vi "auto_alignment_v2-1.vi"() -> ()   [LabVIEW 2024]
uses:
  O:/DSG/Tyler/EIC/DIRC/daq/automated/Thorlabs.MotionControl.IntegratedStepperMotorsCLI.dll
  Thorlabs.MotionControl.IntegratedStepperMotorsCLI.dll
  O:/DSG/Tyler/EIC/DIRC/daq/automated/Thorlabs.MotionControl.Benchtop.StepperMotorCLI.dll
  Thorlabs.MotionControl.Benchtop.StepperMotorCLI.dll
  301acc45-ca86-4456-a934-959b204451cf.vi
  <vilib>/Array/Sort 2D Array - Pop Stack.vi
  <vilib>/Array/Sort 2D Array - Push Stack.vi
  301acc45-ca86-4456-a934-959b204451cf.vi/269d4b3b-47f5-49e3-8884-44851e4dd9d5.vi
  301acc45-ca86-4456-a934-959b204451cf.vi/6d99389c-673d-4efb-bf33-19b32bcf4cf8.vi
  <vilib>/Utility/file.llb/Read Delimited Spreadsheet (string).vi
  <vilib>/gmath/interp.llb/Interpolate 2D Scattered (1D).vi
  <vilib>/gmath/NI_AAL_Interpolation.lvlib
panel:
  out "sim_y-range":dbl[](array[numeric])
  out "sim_x-range":dbl[](array[numeric])
  out "sim_max":dbl[](array[numeric])
  out "Array":string[](array[string])
  in  "early-stop":bool
  out "state":string
  out "nPts":dbl
  out "pt-history":dbl[][](array[numeric])
  out "real-mode":bool
  out "sim-iCorr":dbl[](array[numeric])
  out "sim-pdy":dbl[](array[numeric])
  out "sim-pdx":dbl[](array[numeric])
  out "sim-data":dbl[][](array[numeric])
  out "Final Location":dbl[](array[numeric])
  in  "F=cRIO 2":bool
  out "x_c":dbl[](array[numeric])
  out "x_e":dbl[](array[numeric])
  out "x_r":dbl[](array[numeric])
  out "timeout":bool
  out "se_done":bool
  in  "se_goal":dbl=0.04
  out "squared_error":dbl
  out "x_o":dbl[](array[numeric])
  in  "F=cRIO":bool
  in  "xStart":dbl=265.0 format="%#_13g"
  in  "yStart":dbl=127.5 format="%#_13g"
  out "meter-error-out":errorcluster
  out "stage-error-out":errorcluster
  in  "stage-refs":T1
  in  "stage-error-in":errorcluster
  in  "meter-error-in":errorcluster
  in  "PD Values":cluster{"PD1":dbl, "PD2":dbl, "PD3":dbl}
  in  "nSamples":dbl=10.0 caption="# Samples"
  in  "meter-visa":refnum<visa-resource-name>
  in  "NM-params":T2={"alpha"=1.0, "gamma"=2.0, "rho"=0.5, "sigma"=0.5, "simplex L"=0.5}
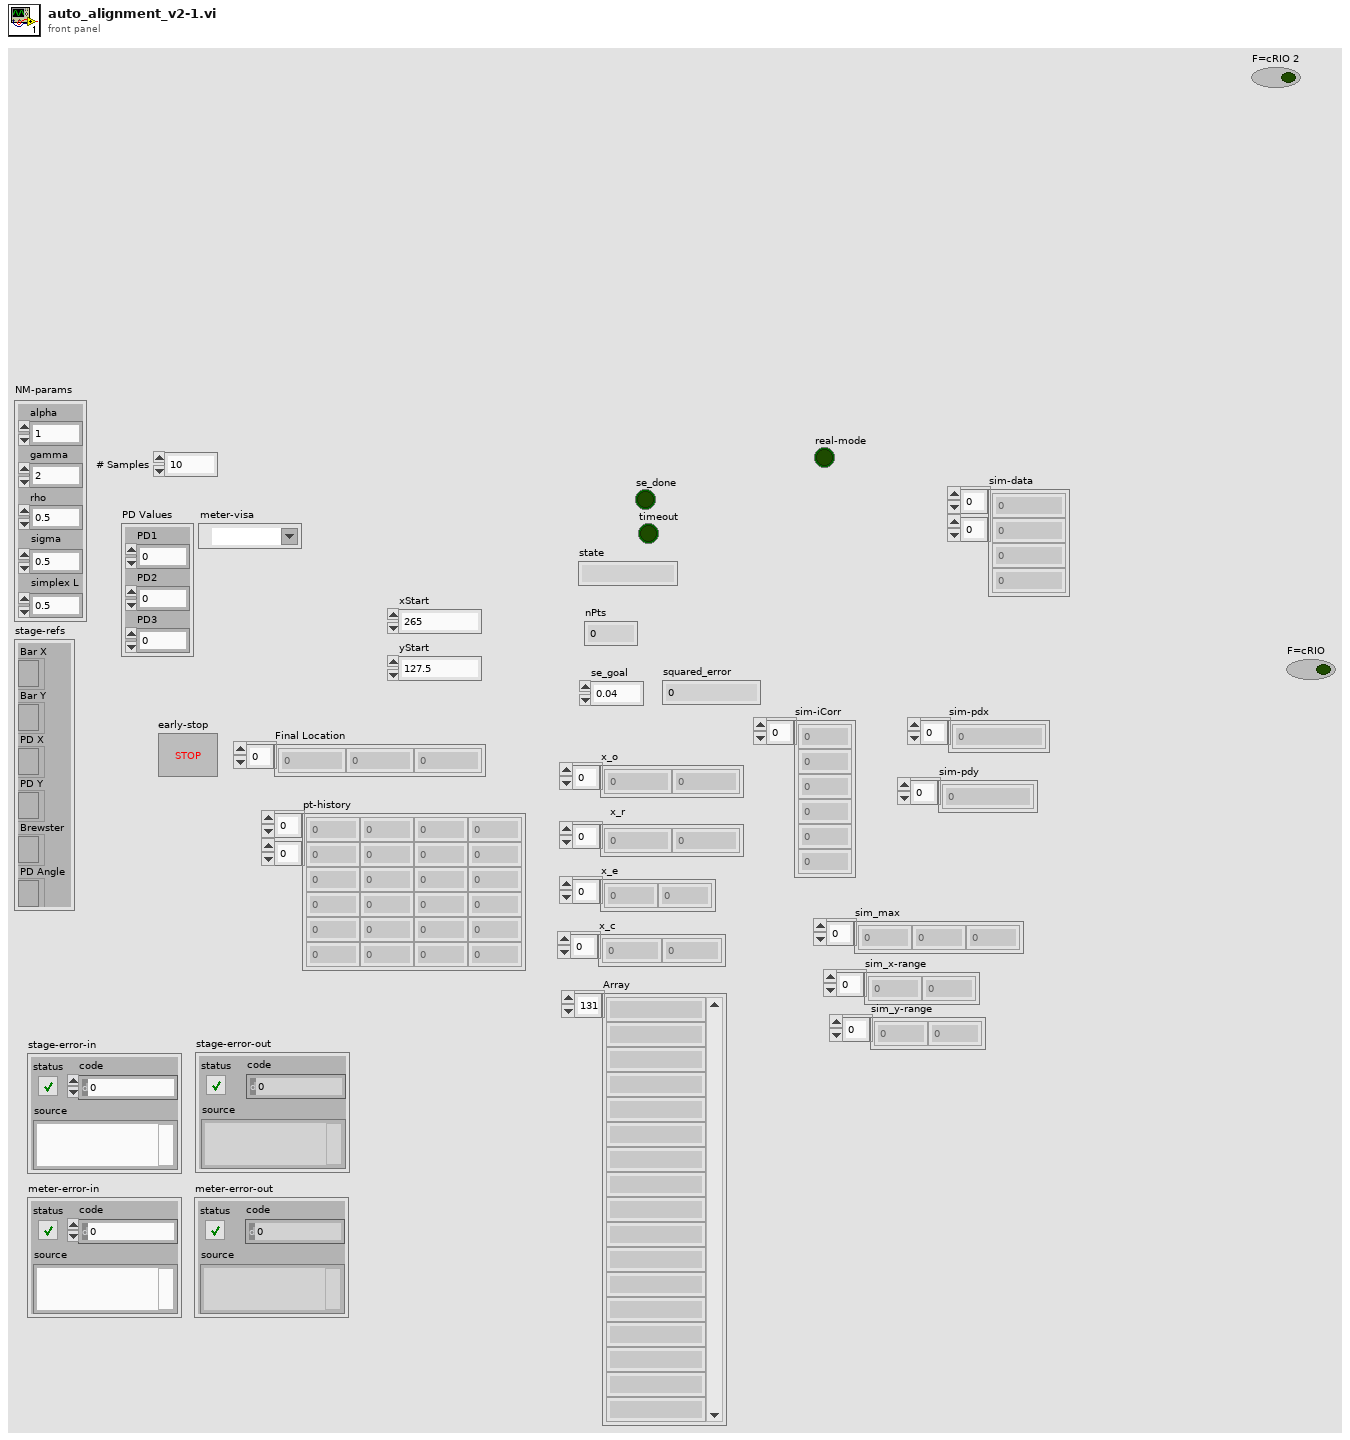
[diagram p1: front panel]
types:
  T1 = cluster{"Bar X":refnum<k24>, "Bar Y":refnum<k24>, "PD X":refnum<k24>, "PD Y":refnum<k24>, "Brewster":refnum<k24>, "PD Angle":refnum<k24>}
  T2 = cluster{"alpha":dbl, "gamma":dbl, "rho":dbl, "sigma":dbl, "simplex L":dbl}
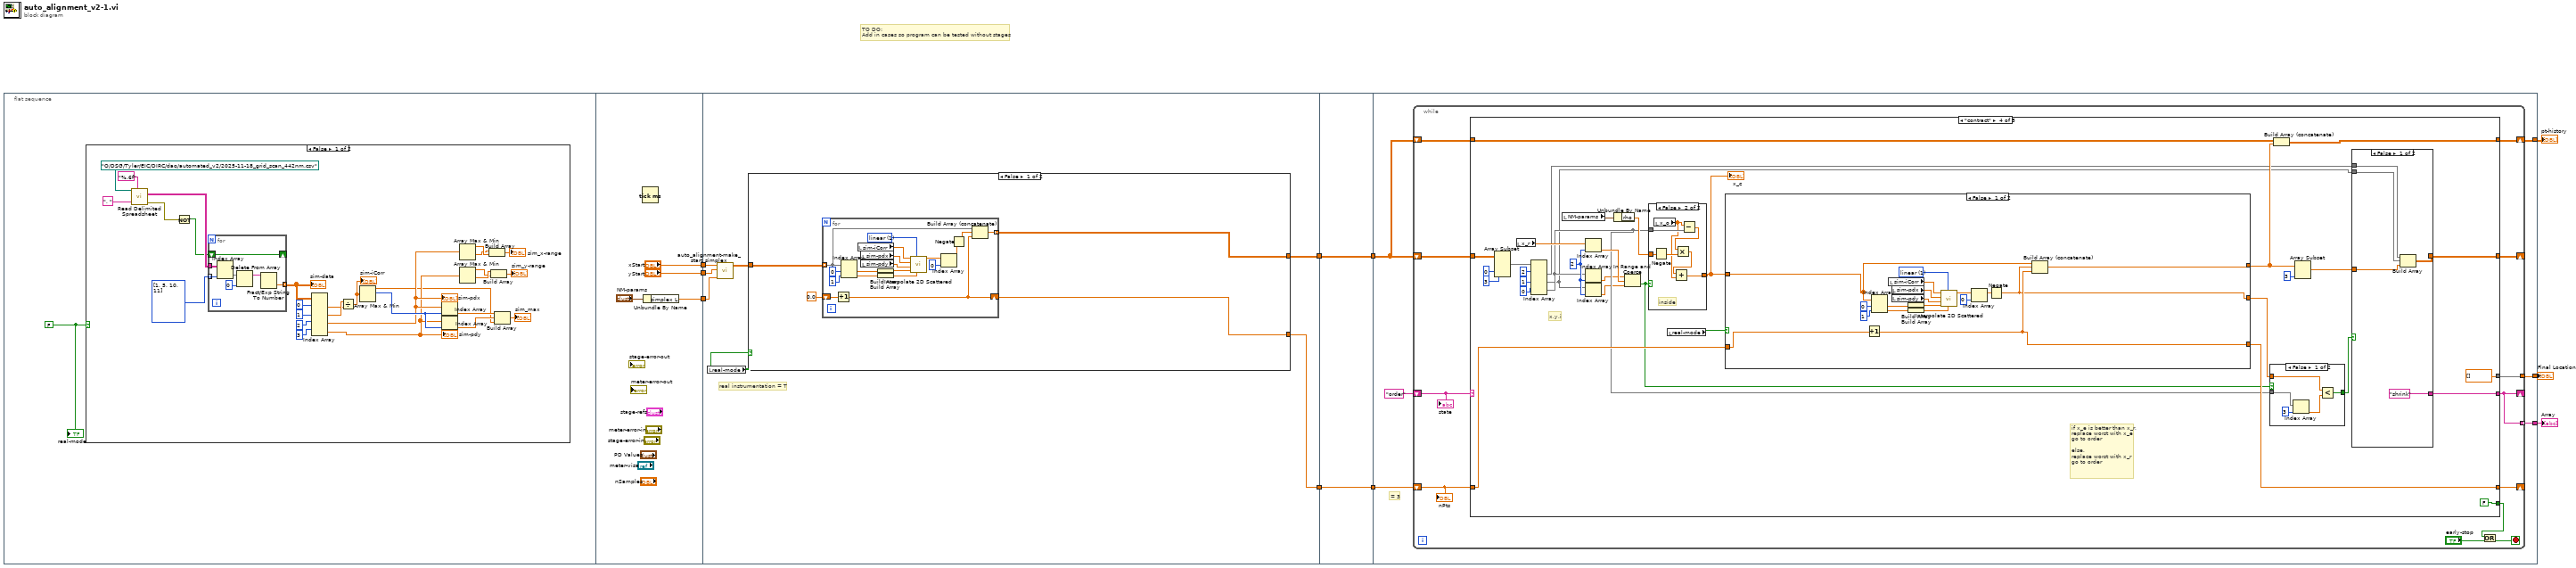
[diagram p0: block diagram]
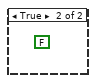
[diagram p2: hidden frame]
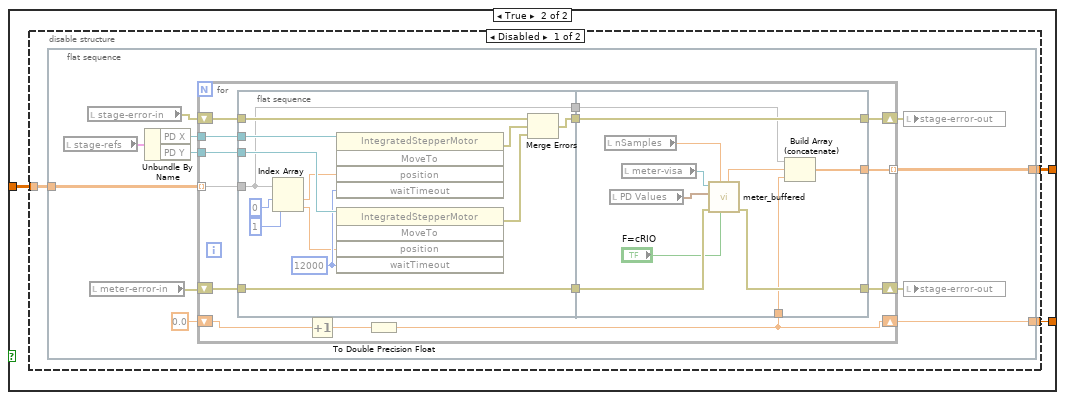
[diagram p3: hidden frame]
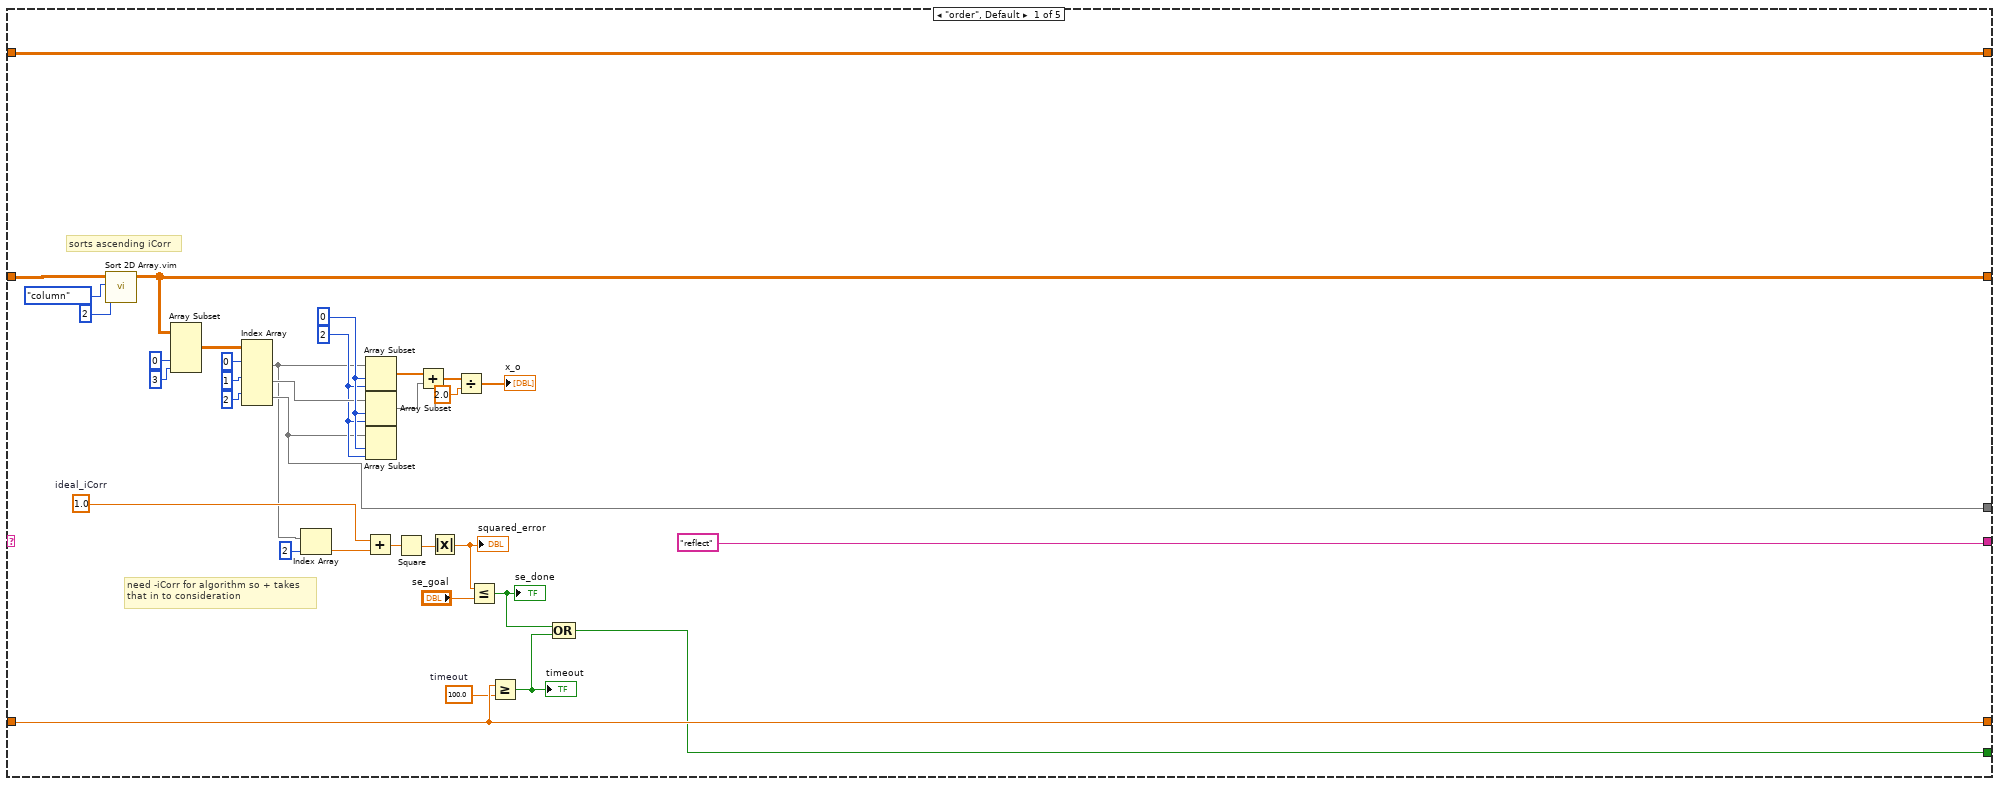
[diagram p5: hidden frame]
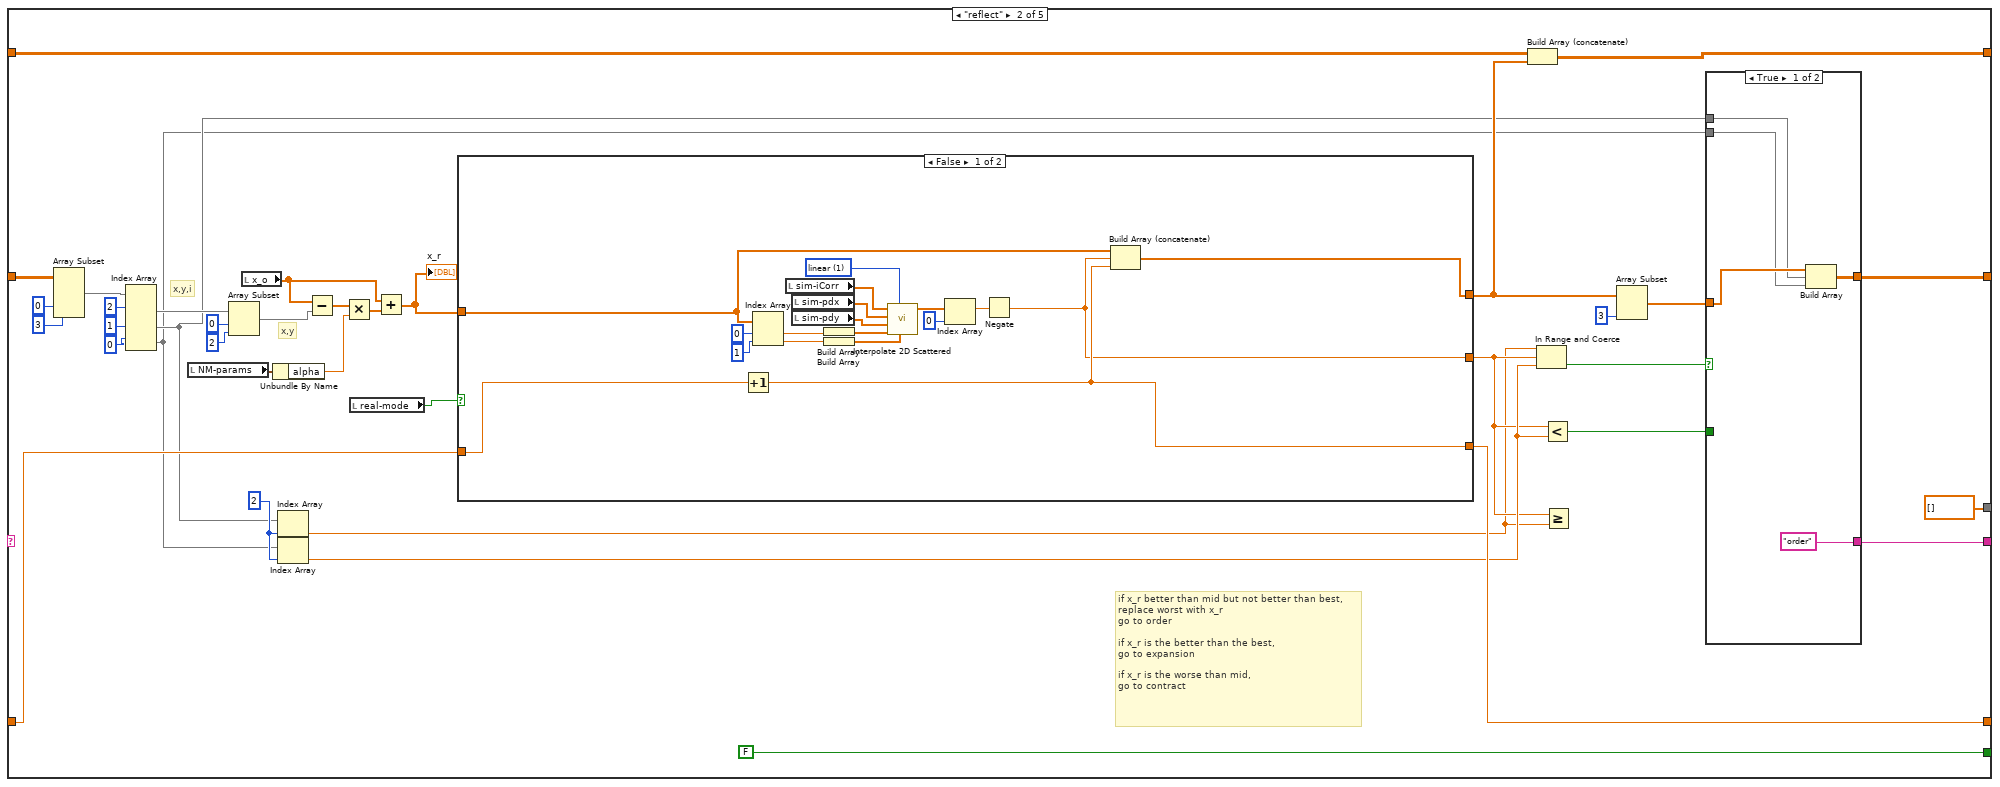
[diagram p6: hidden frame]
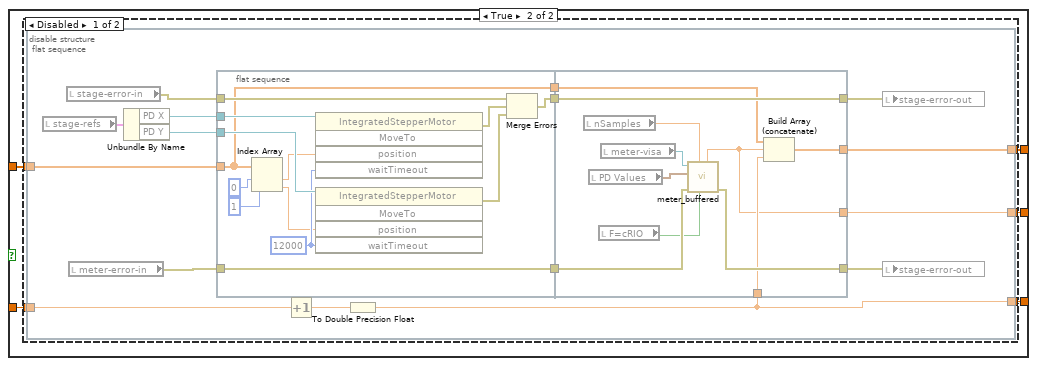
[diagram p7: hidden frame]
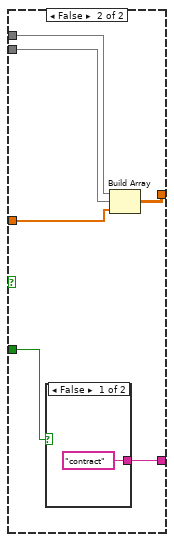
[diagram p9: hidden frame]
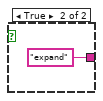
[diagram p10: hidden frame]
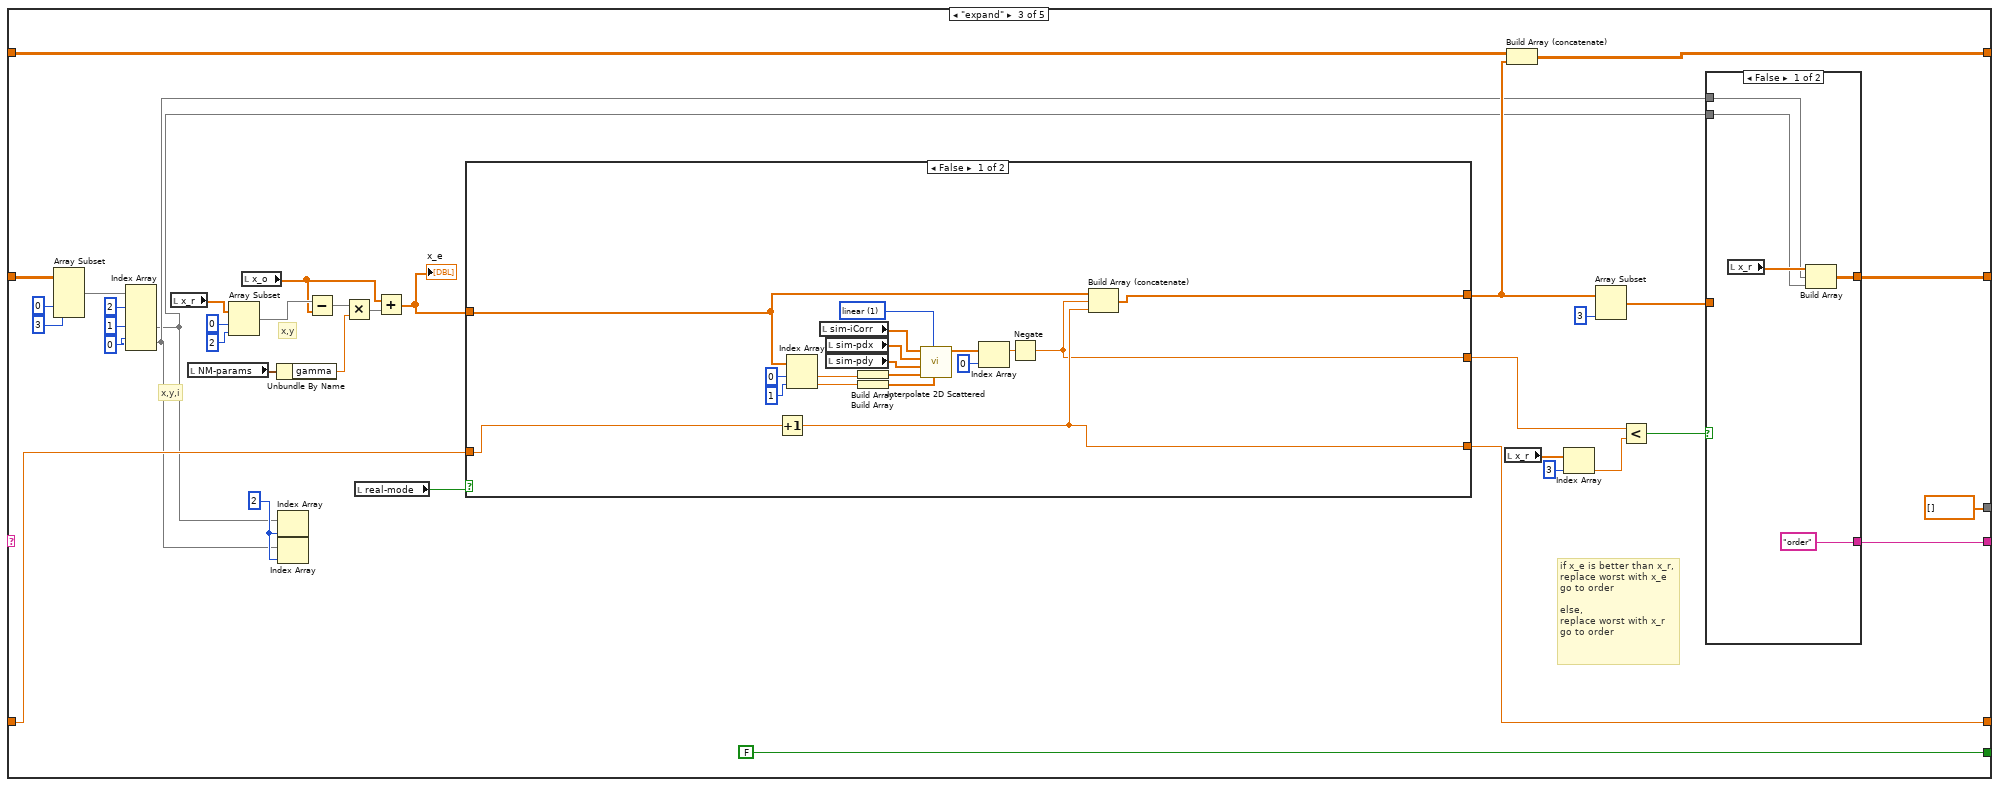
[diagram p11: hidden frame]
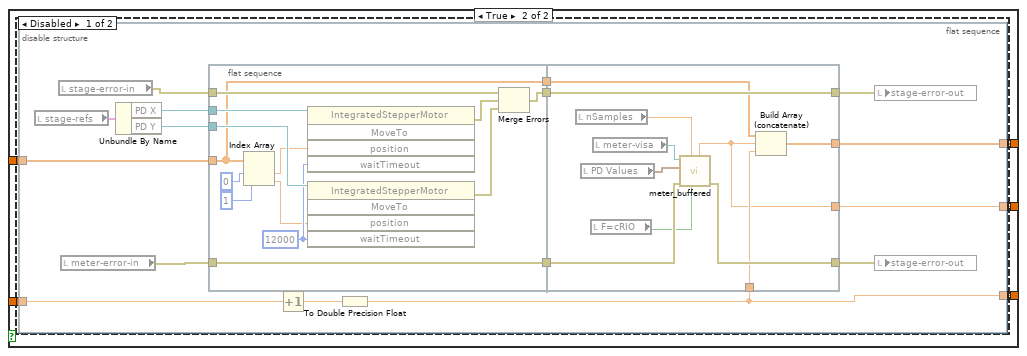
[diagram p12: hidden frame]
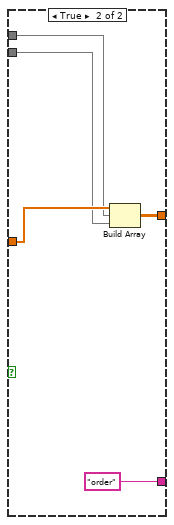
[diagram p14: hidden frame]
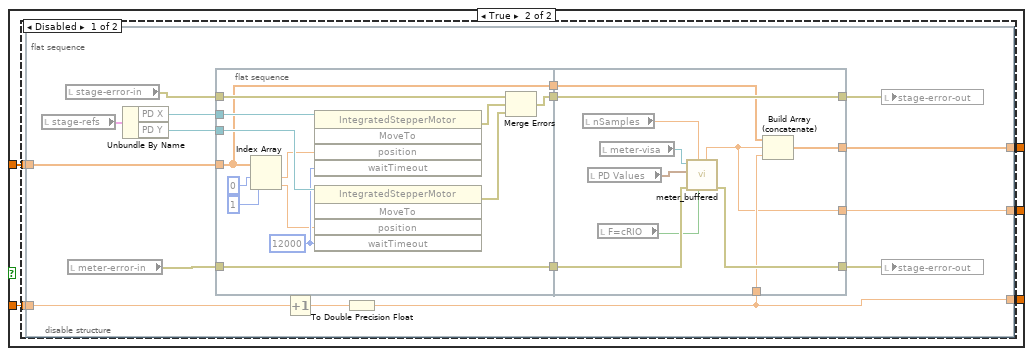
[diagram p15: hidden frame]
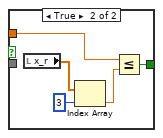
[diagram p17: hidden frame]
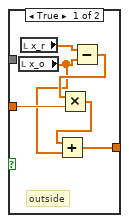
[diagram p18: hidden frame]
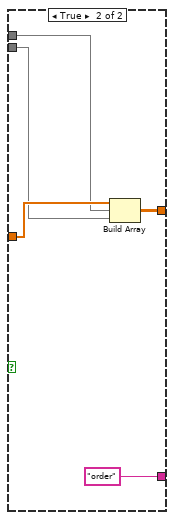
[diagram p19: hidden frame]
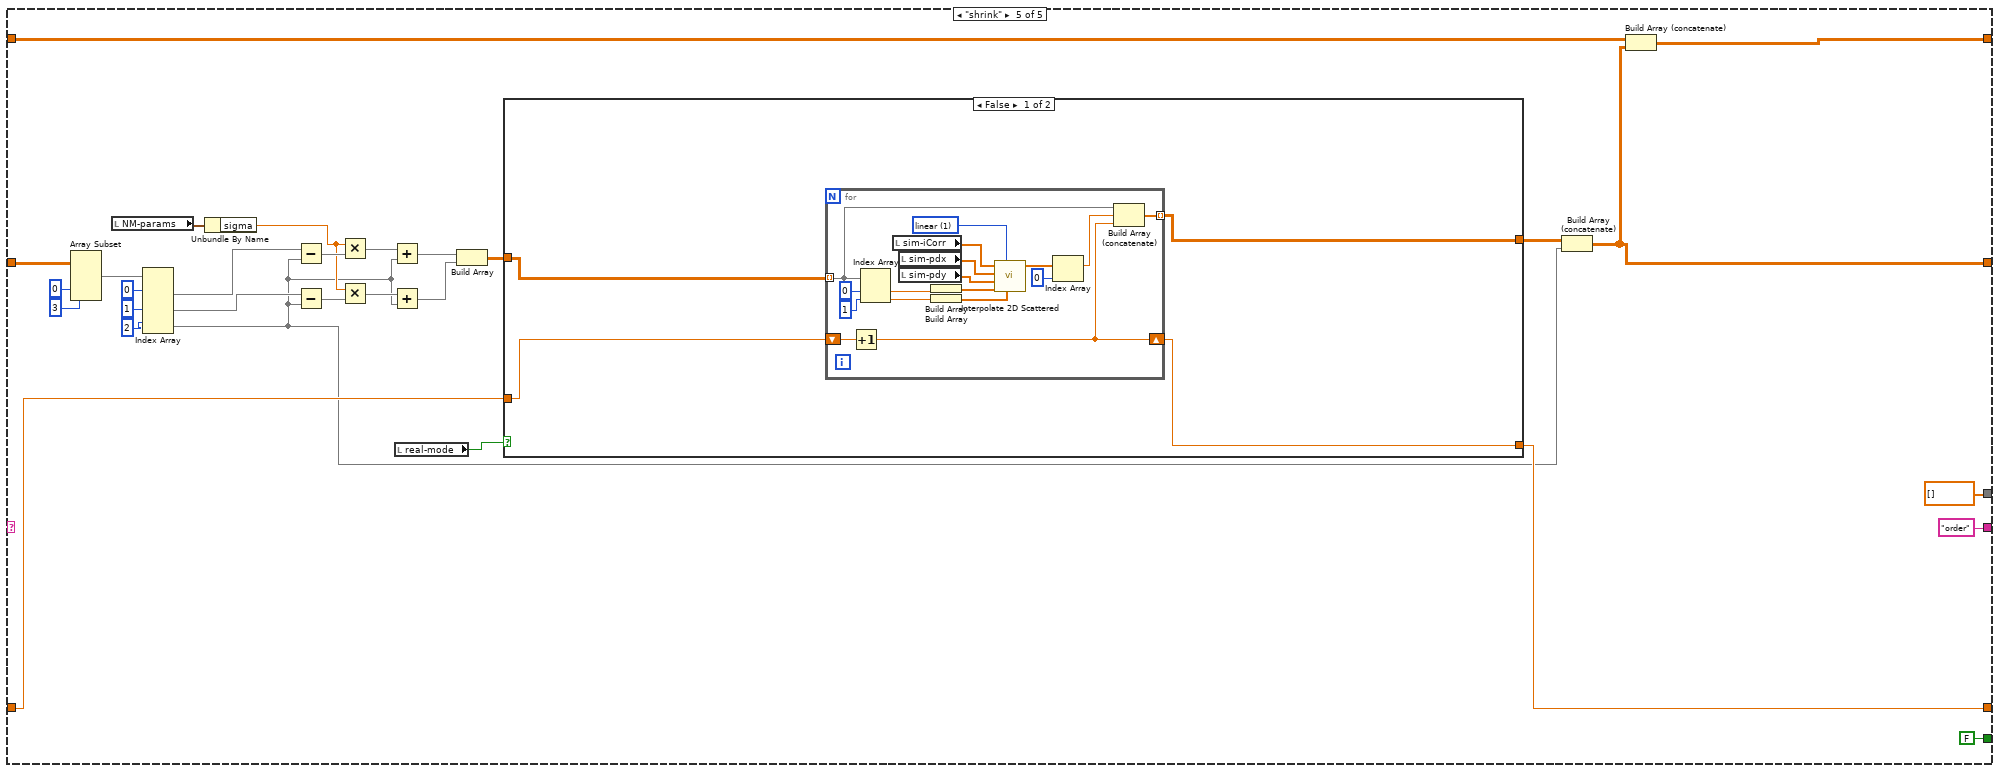
[diagram p20: hidden frame]
diagram:
  # "TO DO:\nAdd in cases so program can be tested without stages"
  n1 = flat-sequence {
    tunnel: ["xStart"] -> w10
    tunnel: ["yStart"] -> w9
    tunnel: [w47] -> w8
    tunnel: w10 -> [w53]
    tunnel: w9 -> [w54]
    tunnel: w8 -> [w55]
    tunnel: [w57] -> w4
    tunnel: [w56] -> w2
    tunnel: w4 -> [w136]
    tunnel: [w136] -> w3
    tunnel: w2 -> [w135]
    tunnel: [w135] -> w1
    tunnel: w3 -> [w140]
    tunnel: w1 -> [w141]
    tunnel: [w139] -> w7
    tunnel: [w138] -> w6
    tunnel: [w137] -> w5
    frame #0 {
      w11 = FALSE
      n2 = case shown="False" w11 {
        frame False {
          n3 = call-poly <vilib>:"Read Delimited Spreadsheet.vi"("file path (dialog if empty)"=path "O:/DSG/Tyler/EIC/DIRC/daq/automated_v2/2025-11-18_grid_scan_442nm.csv", "format (%s)"="%.6f" ("format (%.3f)"), "delimiter (\\t)"=", " ("delimiter (\\t)")) -> ("all rows"=w35:string[][], "error out"=w37:errorcluster)  [unwired: 7 in, 4 out]
          n4 = Not(x=w37) -> (.not. x?=w33:bool)
          n5 = for {
            tunnel: i32[] [1, 5, 10, 11] -> [w45] mode=indexing
            tunnel: w35 -> [w46]
            shift-right: [w44] -> _
            shift-left: w33 -> [w44]
            tunnel: [w40] -> w26 mode=indexing
            n6 = Index Array(array=w46, index (col)=w45) -> (element=w43:string[])  [unwired: 1 in]
            n7 = Delete From Array(array=w43, index=0) -> (array with subset deleted=w41:string[])  [unwired: 1 in, 1 out]
            n8 = Fract/Exp String To Number(string=w41) -> (number=w40:dbl[])  [unwired: 3 in, 1 out]
          }
          "sim-data" <- w26
          n9 = Index Array(array=w26, index (row) #1=0 ("index"), index (row) #2=1 ("index (row)"), index (row) #3=2 ("index (row)"), index (row) #4=3 ("index (row)")) -> (element #1=w27:dbl[], element #2=w28:dbl[], element #3=w21:dbl[], element #4=w20:dbl[])  [unwired: 4 in]
          "sim-pdx" <- w21
          "sim-pdy" <- w20
          n10 = Divide(x=w28, y=w27) -> (x/y=w12:dbl[])
          "sim-iCorr" <- w12
          n11 = Array Max & Min(array=w12) -> (max value=w13:dbl, max index (indices)=w25:i32)  [unwired: 2 out]
          n12 = Index Array(array=w21, index=w25) -> (element=w24:dbl)
          n13 = Index Array(array=w20, index=w25) -> (element=w23:dbl)
          n14 = Array Max & Min(array=w21) -> (max value=w19:dbl, min value=w18:dbl)  [unwired: 2 out]
          n15 = Array Max & Min(array=w20) -> (max value=w15:dbl, min value=w17:dbl)  [unwired: 2 out]
          n16 = Build Array(w18, w19) -> (→"sim_x-range":dbl[])
          n17 = Build Array(w17, w15) -> (→"sim_y-range":dbl[])
          n18 = Build Array(w24, w23, w13) -> (→"sim_max":dbl[])
        }
        frame True {
          (unwired) FALSE
        }
      }
      "real-mode" <- w11
    }
    frame #1 {
      n19 = Tick Count (ms)() -> ()  [unwired: 1 out]
      n20 = Unbundle By Name("NM-params") -> ("simplex L"=w47:dbl)
    }
    frame #2 {
      # "real instrumentation = T"
      n21 = local read "real-mode"() -> (w51:bool)
      n22 = call "auto_alignment-make_start_simplex.vi"("L"=w55, "yStart"=w54, "xStart"=w53) -> ("Array"=w52:dbl[][])  [unwired: 8 in]
      n23 = case shown="False" w51 {
        tunnel: [w58 w82] -> w57
        tunnel: [w60 w81] -> w56
        tunnel: w52 -> [w59 w80]
        frame False {
          n24 = for {
            shift-right: [w63] -> w60
            shift-left: 0.0 -> [w75]
            tunnel: w59 -> [w68] mode=indexing
            tunnel: [w67] -> w58 mode=indexing
            w79 = 1 items=["nearest", "linear", "cubic", "biharmonic spline "] ("method")
            n25 = Increment(x=w75) -> (x+1=w63:dbl)
            n26 = Index Array(array=w68, index #1=0 ("index"), index #2=1 ("index")) -> (element #1=w72:dbl, element #2=w70:dbl)
            n27 = local read "sim-iCorr"() -> (w78:dbl[])
            n28 = local read "sim-pdx"() -> (w77:dbl[])
            n29 = local read "sim-pdy"() -> (w76:dbl[])
            n30 = Build Array(w72) -> (w71:dbl[])
            n31 = Build Array(w70) -> (w69:dbl[])
            n32 = call-poly <vilib>:"Interpolate 2D Scattered.vi"("Yi"=w69, "method"=w79, "Xi"=w71, "Y"=w76, "X"=w77, "Z"=w78) -> ("Zi"=w66:dbl[])  [unwired: 4 in, 1 out]
            n33 = Index Array(array=w66, index=0) -> (element=w65:dbl)
            n34 = Negate(x=w65) -> (-x=w62:dbl)
            n35 = Build Array (concatenate)(w68, w62, w63) -> (w67:dbl[])
          }
        }
        frame True {
          n36 = disable-structure shown="Disabled" {
            disable-tunnel: [w85 _] -> w82
            disable-tunnel: [w84 _] -> w81
            disable-tunnel: w80 -> [w83 _]
            frame Disabled {
              n37 = flat-sequence {
                tunnel: [w94] -> w85
                tunnel: [w88] -> w84
                tunnel: w83 -> [w86]
                frame #0 {
                  n38 = local read "stage-refs"() -> (w90:T1)
                  n39 = local read "stage-error-in"() -> (w91:errorcluster)
                  n40 = local read "meter-error-in"() -> (w89:errorcluster)
                  n41 = Unbundle By Name(w90) -> ("PD X"=w96:refnum<k24>, "PD Y"=w95:refnum<k24>)
                  n42 = for {
                    tunnel: w96 -> [w110]
                    tunnel: w95 -> [w109]
                    tunnel: w86 -> [w106] mode=indexing
                    shift-right: [w104] -> w92
                    shift-left: w91 -> [w108]
                    tunnel: [w107] -> w94 mode=indexing
                    shift-right: [w105] -> w93
                    shift-left: w89 -> [w103]
                    shift-right: [w98] -> w88
                    shift-left: 0.0 -> [w97]
                    n43 = flat-sequence {
                      tunnel: w110 -> [w121]
                      tunnel: w109 -> [w120]
                      tunnel: w108 -> [w114]
                      tunnel: w106 -> [w112]
                      tunnel: w103 -> [w111]
                      tunnel: [w113] -> w102
                      tunnel: [w112] -> w101
                      tunnel: [w111] -> w100
                      tunnel: [w134] -> w104
                      tunnel: [w130] -> w105
                      tunnel: [w133] -> w107
                      tunnel: w102 -> [w134]
                      tunnel: w101 -> [w132]
                      tunnel: w100 -> [w131]
                      tunnel: w98 -> [w124]
                      frame #0 {
                        w119 = 12000 ("waitTimeout")
                        n44 = Index Array(array=w112, index #1=0 ("index"), index #2=1 ("index")) -> (element #1=w116:dbl, element #2=w115:dbl)
                        n45 = invoke class="IntegratedStepperMotor" method="MoveTo"(reference=w121, "position"=w116, "waitTimeout"=w119) -> (error out=w123:errorcluster)  [unwired: 2 in, 4 out]
                        n46 = invoke class="IntegratedStepperMotor" method="MoveTo"(reference=w120, "position"=w115, "waitTimeout"=w119) -> (error out=w122:errorcluster)  [unwired: 2 in, 4 out]
                        n47 = Merge Errors(w114, w123, w122) -> (w113:errorcluster)
                      }
                      frame #1 {
                        n48 = local read "nSamples"() -> (w129:dbl)
                        n49 = local read "PD Values"() -> (w127:cluster{"PD1":dbl, "PD2":dbl, "PD3":dbl})
                        n50 = local read "meter-visa"() -> (w128:refnum<visa-resource-name>)
                        n51 = call "meter_buffered.vi"("F=cRIO"="F=cRIO", "Samples"=w129, "error in"=w131, "PD ranges"=w127, "meter-VISA"=w128) -> ("error out"=w130:errorcluster, "iCorr"=w125:dbl)  [unwired: 2 in, 3 out]
                        n52 = Build Array (concatenate)(w132, w125, w124) -> (w133:dbl[])
                      }
                    }
                    n53 = Increment(x=w97) -> (x+1=w99:dbl)
                    n54 = To Double Precision Float(number=w99) -> (double precision float=w98:dbl)
                  }
                  n55 = local write "stage-error-out"(w92) -> ()
                  n56 = local write "stage-error-out"(w93) -> ()
                }
              }
            }
            frame Enabled {
            }
          }
        }
      }
    }
    frame #3 {
    }
    frame #4 {
      # "= 3"
      n57 = while {
        shift-right: [w148] -> w138
        shift-left: w140 -> [w153]
        shift-right: [w149] -> _
        shift-left: w140 -> [w152]
        shift-right: [w143] -> _
        shift-left: "order" -> [w154]
        shift-right: [w150] -> _
        shift-left: w141 -> [w151]
        tunnel: [w147] -> w139
        tunnel: [w143] -> w137 mode=indexing
        stop <- w145 stop-if-true
        n58 = case shown="\"contract\"" w154 {
          tunnel: w153 -> [w174 w207 w327 w444 w563]
          tunnel: w152 -> [w172 w192 w324 w442 w576]
          tunnel: ["reflect" w203 w322 w440 "order"] -> w143
          tunnel: w151 -> [w163 w209 w329 w446 w564]
          tunnel: [w163 w208 w328 w445 w561] -> w150
          tunnel: [w164 w204 w323 w441 w557] -> w149
          tunnel: [w159 FALSE FALSE FALSE FALSE] -> w144
          tunnel: [w174 w206 w326 w443 w562] -> w148
          tunnel: [w158 dbl[] [] dbl[] [] dbl[] [] dbl[] []] -> w147
          frame "order", Default {
            w162 = 100.0  # timeout
            w169 = 1.0  # ideal_iCorr
            w179 = 2 ("length")
            w181 = 0 ("index")
            # "need -iCorr for algorithm so + takes\nthat in to consideration"
            # "sorts ascending iCorr"
            n59 = call "Sort 2D Array.vim"("index"=2, "dimension to index (column)"=enum16{"column", "row"}."column", "2D array"=w172) -> ("sorted 2D array"=w164:dbl[][])  [unwired: 7 in, 1 out]
            n60 = Array Subset(array=w164, index (col)=0 ("index"), length (col)=3 ("length")) -> (w173:dbl[][])  [unwired: 2 in]
            n61 = Index Array(array=w173, index (row) #1=0 ("index (row)"), index (row) #2=1 ("index (row)"), index (row) #3=2 ("index (row)")) -> (element #1=w155:dbl[], element #2=w180:dbl[], element #3=w158:dbl[])  [unwired: 3 in]
            n62 = Index Array(array=w155, index=2) -> (element=w170:dbl)
            n63 = Add(x=w169, y=w170) -> (x+y=w168:dbl)
            n64 = Array Subset(array=w155, index=w181, length=w179) -> (w157:dbl[])
            n65 = Array Subset(array=w180, index=w181, length=w179) -> (w156:dbl[])
            n66 = Array Subset(array=w158, index=w181, length=w179) -> ()  [unwired: 1 out]
            n67 = Square(x=w168) -> (x^2=w167:dbl)
            n68 = Add(x=w157, y=w156) -> (x+y=w178:dbl[])
            n69 = Absolute Value(x=w167) -> (abs(x)=w166:dbl)
            "squared_error" <- w166
            n70 = Divide(x=w178, y=2.0) -> (x/y=→"x_o":dbl[])
            n71 = Less Or Equal?(x=w166, y="se_goal") -> (x <= y?=w161:bool)
            "se_done" <- w161
            n72 = Greater Or Equal?(x=w163, y=w162) -> (x >= y?=w160:bool)
            "timeout" <- w160
            n73 = Compound Arithmetic op=OR(w161, w160) -> (w159:bool)
          }
          frame "reflect" {
            w205 = 2 ("index")
            # "x,y"
            # "if x_r better than mid but not better than best, \nreplace worst with x_r\ngo to order\n\nif x_r is the better than the best,\ngo to expansion\n\nif x_r is the worse than mid,\ngo to contract"
            # "x,y,i"
            n74 = Array Subset(array=w192, index (col)=0 ("index"), length (col)=3 ("length")) -> (w191:dbl[][])  [unwired: 2 in]
            n75 = Index Array(array=w191, index (row) #1=2 ("index (row)"), index (row) #2=1 ("index (row)"), index (row) #3=0 ("index (row)")) -> (element #1=w219:dbl[], element #2=w190:dbl[], element #3=w189:dbl[])  [unwired: 3 in]
            n76 = local read "NM-params"() -> (w216:T2)
            n77 = Array Subset(array=w219, index=0 ("index (row)"), length=2 ("index (row)")) -> (w215:dbl[])
            n78 = local read "x_o"() -> (w212:dbl[])
            n79 = Unbundle By Name(w216) -> ("alpha"=w213:dbl)
            n80 = Index Array(array=w190, index=w205) -> (element=w194:dbl)
            n81 = Index Array(array=w189, index=w205) -> (element=w197:dbl)
            n82 = Subtract(x=w212, y=w215) -> (x-y=w214:dbl[])
            n83 = Multiply(x=w214, y=w213) -> (x*y=w211:dbl[])
            n84 = local read "real-mode"() -> (w198:bool)
            n85 = Add(x=w212, y=w211) -> (x+y=w210:dbl[])
            "x_r" <- w210
            n86 = case shown="False" w198 {
              tunnel: w210 -> [w231 w248]
              tunnel: w209 -> [w230 w247]
              tunnel: [w229 w246] -> w208
              tunnel: [w226 w245] -> w195
              tunnel: [w227 w244] -> w202
              frame False {
                w243 = 1 items=["nearest", "linear", "cubic", "biharmonic spline "] ("method")
                n87 = Increment(x=w230) -> (x+1=w229:dbl)
                n88 = Index Array(array=w231, index #1=0 ("index"), index #2=1 ("index")) -> (element #1=w237:dbl, element #2=w235:dbl)
                n89 = local read "sim-iCorr"() -> (w242:dbl[])
                n90 = local read "sim-pdx"() -> (w241:dbl[])
                n91 = local read "sim-pdy"() -> (w240:dbl[])
                n92 = Build Array(w237) -> (w236:dbl[])
                n93 = Build Array(w235) -> (w234:dbl[])
                n94 = call-poly <vilib>:"Interpolate 2D Scattered.vi"("Yi"=w234, "method"=w243, "Xi"=w236, "Y"=w240, "X"=w241, "Z"=w242) -> ("Zi"=w233:dbl[])  [unwired: 4 in, 1 out]
                n95 = Index Array(array=w233, index=0) -> (element=w228:dbl)
                n96 = Negate(x=w228) -> (-x=w226:dbl)
                n97 = Build Array (concatenate)(w231, w226, w229) -> (w227:dbl[])
              }
              frame True {
                n98 = disable-structure shown="Disabled" {
                  disable-tunnel: w248 -> [w253 _]
                  disable-tunnel: w247 -> [w252 _]
                  disable-tunnel: [w251 _] -> w246
                  disable-tunnel: [w250 _] -> w245
                  disable-tunnel: [w249 _] -> w244
                  frame Disabled {
                    n99 = flat-sequence {
                      tunnel: [w267] -> w249
                      tunnel: [w261] -> w251
                      tunnel: w253 -> [w260]
                      tunnel: w252 -> [w255]
                      tunnel: [w254] -> w250
                      frame #0 {
                        n100 = local read "stage-refs"() -> (w263:T1)
                        n101 = local read "stage-error-in"() -> (w264:errorcluster)
                        n102 = local read "meter-error-in"() -> (w262:errorcluster)
                        n103 = Unbundle By Name(w263) -> ("PD X"=w269:refnum<k24>, "PD Y"=w268:refnum<k24>)
                        n104 = flat-sequence {
                          tunnel: w269 -> [w280]
                          tunnel: w268 -> [w279]
                          tunnel: w264 -> [w273]
                          tunnel: w260 -> [w271]
                          tunnel: w262 -> [w270]
                          tunnel: [w272] -> w259
                          tunnel: [w271] -> w258
                          tunnel: [w270] -> w257
                          tunnel: [w293] -> w265
                          tunnel: [w289] -> w266
                          tunnel: [w292] -> w267
                          tunnel: w259 -> [w293]
                          tunnel: w258 -> [w291]
                          tunnel: w257 -> [w290]
                          tunnel: w261 -> [w285]
                          tunnel: [w284] -> w254
                          frame #0 {
                            w278 = 12000 ("waitTimeout")
                            n105 = Index Array(array=w271, index #1=0 ("index"), index #2=1 ("index")) -> (element #1=w275:dbl, element #2=w274:dbl)
                            n106 = invoke class="IntegratedStepperMotor" method="MoveTo"(reference=w280, "position"=w275, "waitTimeout"=w278) -> (error out=w282:errorcluster)  [unwired: 2 in, 4 out]
                            n107 = invoke class="IntegratedStepperMotor" method="MoveTo"(reference=w279, "position"=w274, "waitTimeout"=w278) -> (error out=w281:errorcluster)  [unwired: 2 in, 4 out]
                            n108 = Merge Errors(w273, w282, w281) -> (w272:errorcluster)
                          }
                          frame #1 {
                            n109 = local read "nSamples"() -> (w288:dbl)
                            n110 = local read "PD Values"() -> (w286:cluster{"PD1":dbl, "PD2":dbl, "PD3":dbl})
                            n111 = local read "F=cRIO"() -> (w283:bool)
                            n112 = local read "meter-visa"() -> (w287:refnum<visa-resource-name>)
                            n113 = call "meter_buffered.vi"("F=cRIO"=w283, "Samples"=w288, "error in"=w290, "PD ranges"=w286, "meter-VISA"=w287) -> ("error out"=w289:errorcluster, "iCorr"=w284:dbl)  [unwired: 2 in, 3 out]
                            n114 = Build Array (concatenate)(w291, w284, w285) -> (w292:dbl[])
                          }
                        }
                        n115 = Increment(x=w255) -> (x+1=w256:dbl)
                        n116 = To Double Precision Float(number=w256) -> (double precision float=w261:dbl)
                        n117 = local write "stage-error-out"(w265) -> ()
                        n118 = local write "stage-error-out"(w266) -> ()
                      }
                    }
                  }
                  frame Enabled {
                  }
                }
              }
            }
            n119 = Build Array (concatenate)(w207, w202) -> (w206:dbl[][])
            n120 = In Range and Coerce(upper limit=w194, x=w195, lower limit=w197) -> (In Range?=w196:bool)  [unwired: 1 out]
            n121 = Less?(x=w195, y=w197) -> (x < y?=w193:bool)
            n122 = Greater Or Equal?(x=w195, y=w194) -> ()  [unwired: 1 out]
            n123 = Array Subset(array=w202, length=3) -> (w200:dbl[])  [unwired: 1 in]
            n124 = case shown="True" w196 {
              tunnel: [w297 w302] -> w204
              tunnel: ["order" w304] -> w203
              tunnel: w200 -> [w298 w299]
              tunnel: w193 -> [_ w303]
              tunnel: w190 -> [w295 w301]
              tunnel: w189 -> [w294 w300]
              frame True {
                n125 = Build Array(w298, w295, w294) -> (w297:dbl[][])
              }
              frame False {
                n126 = case shown="False" w303 {
                  tunnel: ["contract" "expand"] -> w304
                  frame False {
                  }
                  frame True {
                  }
                }
                n127 = Build Array(w301, w300, w299) -> (w302:dbl[][])
              }
            }
          }
          frame "expand" {
            w325 = 2 ("index")
            # "x,y"
            # "if x_e is better than x_r,\nreplace worst with x_e\ngo to order\n\nelse,\nreplace worst with x_r\ngo to order"
            # "x,y,i"
            n128 = Array Subset(array=w324, index (col)=0 ("index"), length (col)=3 ("length")) -> (w342:dbl[][])  [unwired: 2 in]
            n129 = Index Array(array=w342, index (row) #1=2 ("index (row)"), index (row) #2=1 ("index (row)"), index (row) #3=0 ("index (row)")) -> (element #2=w307:dbl[], element #3=w308:dbl[])  [unwired: 3 in, 1 out]
            n130 = local read "x_r"() -> (w318:dbl[])
            n131 = local read "NM-params"() -> (w334:T2)
            n132 = Array Subset(array=w318, index=0 ("index (row)"), length=2 ("index (row)")) -> (w310:dbl[])
            n133 = local read "x_o"() -> (w309:dbl[])
            n134 = Unbundle By Name(w334) -> ("gamma"=w332:dbl)
            n135 = Index Array(array=w307, index=w325) -> ()  [unwired: 1 out]
            n136 = Index Array(array=w308, index=w325) -> ()  [unwired: 1 out]
            n137 = Subtract(x=w310, y=w309) -> (x-y=w333:dbl[])
            n138 = Multiply(x=w333, y=w332) -> (x*y=w331:dbl[])
            n139 = local read "real-mode"() -> (w311:bool)
            n140 = Add(x=w309, y=w331) -> (x+y=w330:dbl[])
            "x_e" <- w330
            n141 = case shown="False" w311 {
              tunnel: w330 -> [w349 w366]
              tunnel: w329 -> [w348 w365]
              tunnel: [w347 w364] -> w328
              tunnel: [w346 w363] -> w321
              tunnel: [w344 w362] -> w316
              frame False {
                w361 = 1 items=["nearest", "linear", "cubic", "biharmonic spline "] ("method")
                n142 = Increment(x=w348) -> (x+1=w347:dbl)
                n143 = Index Array(array=w349, index #1=0 ("index"), index #2=1 ("index")) -> (element #1=w355:dbl, element #2=w353:dbl)
                n144 = local read "sim-iCorr"() -> (w360:dbl[])
                n145 = local read "sim-pdx"() -> (w359:dbl[])
                n146 = local read "sim-pdy"() -> (w358:dbl[])
                n147 = Build Array(w355) -> (w354:dbl[])
                n148 = Build Array(w353) -> (w352:dbl[])
                n149 = call-poly <vilib>:"Interpolate 2D Scattered.vi"("Yi"=w352, "method"=w361, "Xi"=w354, "Y"=w358, "X"=w359, "Z"=w360) -> ("Zi"=w351:dbl[])  [unwired: 4 in, 1 out]
                n150 = Index Array(array=w351, index=0) -> (element=w345:dbl)
                n151 = Negate(x=w345) -> (-x=w344:dbl)
                n152 = Build Array (concatenate)(w349, w344, w347) -> (w346:dbl[])
              }
              frame True {
                n153 = disable-structure shown="Disabled" {
                  disable-tunnel: w366 -> [w371 _]
                  disable-tunnel: w365 -> [w370 _]
                  disable-tunnel: [w369 _] -> w364
                  disable-tunnel: [w368 _] -> w363
                  disable-tunnel: [w367 _] -> w362
                  frame Disabled {
                    n154 = flat-sequence {
                      tunnel: [w385] -> w368
                      tunnel: [w379] -> w369
                      tunnel: w371 -> [w378]
                      tunnel: w370 -> [w373]
                      tunnel: [w372] -> w367
                      frame #0 {
                        n155 = local read "stage-refs"() -> (w381:T1)
                        n156 = local read "stage-error-in"() -> (w382:errorcluster)
                        n157 = local read "meter-error-in"() -> (w380:errorcluster)
                        n158 = Unbundle By Name(w381) -> ("PD X"=w387:refnum<k24>, "PD Y"=w386:refnum<k24>)
                        n159 = flat-sequence {
                          tunnel: w387 -> [w398]
                          tunnel: w386 -> [w397]
                          tunnel: w382 -> [w391]
                          tunnel: w378 -> [w389]
                          tunnel: w380 -> [w388]
                          tunnel: [w390] -> w377
                          tunnel: [w389] -> w376
                          tunnel: [w388] -> w375
                          tunnel: [w411] -> w383
                          tunnel: [w407] -> w384
                          tunnel: [w410] -> w385
                          tunnel: w377 -> [w411]
                          tunnel: w376 -> [w409]
                          tunnel: w375 -> [w408]
                          tunnel: w379 -> [w403]
                          tunnel: [w402] -> w372
                          frame #0 {
                            w396 = 12000 ("waitTimeout")
                            n160 = Index Array(array=w389, index #1=0 ("index"), index #2=1 ("index")) -> (element #1=w393:dbl, element #2=w392:dbl)
                            n161 = invoke class="IntegratedStepperMotor" method="MoveTo"(reference=w398, "position"=w393, "waitTimeout"=w396) -> (error out=w400:errorcluster)  [unwired: 2 in, 4 out]
                            n162 = invoke class="IntegratedStepperMotor" method="MoveTo"(reference=w397, "position"=w392, "waitTimeout"=w396) -> (error out=w399:errorcluster)  [unwired: 2 in, 4 out]
                            n163 = Merge Errors(w391, w400, w399) -> (w390:errorcluster)
                          }
                          frame #1 {
                            n164 = local read "nSamples"() -> (w406:dbl)
                            n165 = local read "PD Values"() -> (w404:cluster{"PD1":dbl, "PD2":dbl, "PD3":dbl})
                            n166 = local read "F=cRIO"() -> (w401:bool)
                            n167 = local read "meter-visa"() -> (w405:refnum<visa-resource-name>)
                            n168 = call "meter_buffered.vi"("F=cRIO"=w401, "Samples"=w406, "error in"=w408, "PD ranges"=w404, "meter-VISA"=w405) -> ("error out"=w407:errorcluster, "iCorr"=w402:dbl)  [unwired: 2 in, 3 out]
                            n169 = Build Array (concatenate)(w409, w402, w403) -> (w410:dbl[])
                          }
                        }
                        n170 = Increment(x=w373) -> (x+1=w374:dbl)
                        n171 = To Double Precision Float(number=w374) -> (double precision float=w379:dbl)
                        n172 = local write "stage-error-out"(w383) -> ()
                        n173 = local write "stage-error-out"(w384) -> ()
                      }
                    }
                  }
                  frame Enabled {
                  }
                }
              }
            }
            n174 = local read "x_r"() -> (w315:dbl[])
            n175 = Build Array (concatenate)(w327, w321) -> (w326:dbl[][])
            n176 = Index Array(array=w315, index=3) -> (element=w313:dbl)
            n177 = Array Subset(array=w321, length=3) -> (w319:dbl[])  [unwired: 1 in]
            n178 = Less?(x=w316, y=w313) -> (x < y?=w317:bool)
            n179 = case shown="False" w317 {
              tunnel: [w416 w420] -> w323
              tunnel: ["order" "order"] -> w322
              tunnel: w319 -> [_ w421]
              tunnel: w308 -> [w413 w418]
              tunnel: w307 -> [w412 w417]
              frame False {
                n180 = local read "x_r"() -> (w414:dbl[])
                n181 = Build Array(w414, w413, w412) -> (w416:dbl[][])
              }
              frame True {
                n182 = Build Array(w421, w418, w417) -> (w420:dbl[][])
              }
            }
          }
          frame "contract" {
            w436 = 2 ("index")
            # "if x_e is better than x_r,\nreplace worst with x_e\ngo to order\n\nelse,\nreplace worst with x_r\ngo to order"
            # "x,y,i"
            n183 = Array Subset(array=w442, index (col)=0 ("index"), length (col)=3 ("length")) -> (w453:dbl[][])  [unwired: 2 in]
            n184 = local read "x_r"() -> (w434:dbl[])
            n185 = Index Array(array=w453, index (row) #1=2 ("index (row)"), index (row) #2=1 ("index (row)"), index (row) #3=0 ("index (row)")) -> (element #1=w423:dbl[], element #2=w422:dbl[], element #3=w428:dbl[])  [unwired: 3 in]
            n186 = local read "NM-params"() -> (w447:T2)
            n187 = Index Array(array=w434, index=w436) -> (element=w435:dbl)
            n188 = Index Array(array=w428, index=w436) -> (element=w426:dbl)
            n189 = Index Array(array=w422, index=w436) -> (element=w427:dbl)
            n190 = Unbundle By Name(w447) -> ("rho"=w433:dbl)
            n191 = In Range and Coerce(upper limit=w426, x=w435, lower limit=w427) -> (In Range?=w431:bool)  [unwired: 1 out]
            n192 = case shown="False" w431 {
              tunnel: w433 -> [w536 w544]
              tunnel: [w533 w542] -> w432
              tunnel: w428 -> [_ w541]
              frame True {
                # "outside"
                n193 = local read "x_o"() -> (w534:dbl[])
                n194 = local read "x_r"() -> (w538:dbl[])
                n195 = Subtract(x=w538, y=w534) -> (x-y=w537:dbl[])
                n196 = Multiply(x=w537, y=w536) -> (x*y=w535:dbl[])
                n197 = Add(x=w535, y=w534) -> (x+y=w533:dbl[])
              }
              frame False {
                # "inside"
                n198 = Negate(x=w544) -> (-x=w540:dbl)
                n199 = local read "x_o"() -> (w539:dbl[])
                n200 = Subtract(x=w539, y=w541) -> (x-y=w545:dbl[])
                n201 = Multiply(x=w545, y=w540) -> (x*y=w543:dbl[])
                n202 = Add(x=w543, y=w539) -> (x+y=w542:dbl[])
              }
            }
            "x_c" <- w432
            n203 = local read "real-mode"() -> (w429:bool)
            n204 = case shown="False" w429 {
              tunnel: w446 -> [w459 w477]
              tunnel: [w458 w476] -> w445
              tunnel: [w456 w475] -> w439
              tunnel: [w455 w474] -> w425
              tunnel: w432 -> [w460 w473]
              frame False {
                w472 = 1 items=["nearest", "linear", "cubic", "biharmonic spline "] ("method")
                n205 = Increment(x=w459) -> (x+1=w458:dbl)
                n206 = Index Array(array=w460, index #1=0 ("index"), index #2=1 ("index")) -> (element #1=w466:dbl, element #2=w464:dbl)
                n207 = local read "sim-iCorr"() -> (w471:dbl[])
                n208 = local read "sim-pdx"() -> (w470:dbl[])
                n209 = local read "sim-pdy"() -> (w469:dbl[])
                n210 = Build Array(w466) -> (w465:dbl[])
                n211 = Build Array(w464) -> (w463:dbl[])
                n212 = call-poly <vilib>:"Interpolate 2D Scattered.vi"("Yi"=w463, "method"=w472, "Xi"=w465, "Y"=w469, "X"=w470, "Z"=w471) -> ("Zi"=w462:dbl[])  [unwired: 4 in, 1 out]
                n213 = Index Array(array=w462, index=0) -> (element=w457:dbl)
                n214 = Negate(x=w457) -> (-x=w455:dbl)
                n215 = Build Array (concatenate)(w460, w455, w458) -> (w456:dbl[])
              }
              frame True {
                n216 = disable-structure shown="Disabled" {
                  disable-tunnel: w477 -> [w482 _]
                  disable-tunnel: [w481 _] -> w476
                  disable-tunnel: [w480 _] -> w475
                  disable-tunnel: [w479 _] -> w474
                  disable-tunnel: w473 -> [w478 _]
                  frame Disabled {
                    n217 = flat-sequence {
                      tunnel: [w496] -> w480
                      tunnel: [w490] -> w481
                      tunnel: w478 -> [w489]
                      tunnel: w482 -> [w484]
                      tunnel: [w483] -> w479
                      frame #0 {
                        n218 = local read "stage-refs"() -> (w492:T1)
                        n219 = local read "stage-error-in"() -> (w493:errorcluster)
                        n220 = local read "meter-error-in"() -> (w491:errorcluster)
                        n221 = Unbundle By Name(w492) -> ("PD X"=w498:refnum<k24>, "PD Y"=w497:refnum<k24>)
                        n222 = flat-sequence {
                          tunnel: w498 -> [w509]
                          tunnel: w497 -> [w508]
                          tunnel: w493 -> [w502]
                          tunnel: w489 -> [w500]
                          tunnel: w491 -> [w499]
                          tunnel: [w501] -> w488
                          tunnel: [w500] -> w487
                          tunnel: [w499] -> w486
                          tunnel: [w522] -> w494
                          tunnel: [w518] -> w495
                          tunnel: [w521] -> w496
                          tunnel: w488 -> [w522]
                          tunnel: w487 -> [w520]
                          tunnel: w486 -> [w519]
                          tunnel: w490 -> [w514]
                          tunnel: [w513] -> w483
                          frame #0 {
                            w507 = 12000 ("waitTimeout")
                            n223 = Index Array(array=w500, index #1=0 ("index"), index #2=1 ("index")) -> (element #1=w504:dbl, element #2=w503:dbl)
                            n224 = invoke class="IntegratedStepperMotor" method="MoveTo"(reference=w509, "position"=w504, "waitTimeout"=w507) -> (error out=w511:errorcluster)  [unwired: 2 in, 4 out]
                            n225 = invoke class="IntegratedStepperMotor" method="MoveTo"(reference=w508, "position"=w503, "waitTimeout"=w507) -> (error out=w510:errorcluster)  [unwired: 2 in, 4 out]
                            n226 = Merge Errors(w502, w511, w510) -> (w501:errorcluster)
                          }
                          frame #1 {
                            n227 = local read "nSamples"() -> (w517:dbl)
                            n228 = local read "PD Values"() -> (w515:cluster{"PD1":dbl, "PD2":dbl, "PD3":dbl})
                            n229 = local read "F=cRIO"() -> (w512:bool)
                            n230 = local read "meter-visa"() -> (w516:refnum<visa-resource-name>)
                            n231 = call "meter_buffered.vi"("F=cRIO"=w512, "Samples"=w517, "error in"=w519, "PD ranges"=w515, "meter-VISA"=w516) -> ("error out"=w518:errorcluster, "iCorr"=w513:dbl)  [unwired: 2 in, 3 out]
                            n232 = Build Array (concatenate)(w520, w513, w514) -> (w521:dbl[])
                          }
                        }
                        n233 = Increment(x=w484) -> (x+1=w485:dbl)
                        n234 = To Double Precision Float(number=w485) -> (double precision float=w490:dbl)
                        n235 = local write "stage-error-out"(w494) -> ()
                        n236 = local write "stage-error-out"(w495) -> ()
                      }
                    }
                  }
                  frame Enabled {
                  }
                }
              }
            }
            n237 = case shown="False" w431 {
              tunnel: w428 -> [w526 _]
              tunnel: w425 -> [w524 w530]
              tunnel: [w525 w528] -> w424
              frame False {
                n238 = Index Array(array=w526, index=3) -> (element=w523:dbl)
                n239 = Less?(x=w524, y=w523) -> (x < y?=w525:bool)
              }
              frame True {
                n240 = local read "x_r"() -> (w531:dbl[])
                n241 = Index Array(array=w531, index=3) -> (element=w529:dbl)
                n242 = Less Or Equal?(x=w530, y=w529) -> (x <= y?=w528:bool)
              }
            }
            n243 = Build Array (concatenate)(w444, w439) -> (w443:dbl[][])
            n244 = Array Subset(array=w439, length=3) -> (w437:dbl[])  [unwired: 1 in]
            n245 = case shown="False" w424 {
              tunnel: [w549 w554] -> w441
              tunnel: ["shrink" "order"] -> w440
              tunnel: w437 -> [w548 w555]
              tunnel: w423 -> [w547 w552]
              tunnel: w422 -> [w546 w551]
              frame False {
                n246 = Build Array(w547, w546, w548) -> (w549:dbl[][])
              }
              frame True {
                n247 = Build Array(w555, w552, w551) -> (w554:dbl[][])
              }
            }
          }
          frame "shrink" {
            n248 = Array Subset(array=w576, index (col)=0 ("index"), length (col)=3 ("length")) -> (w582:dbl[][])  [unwired: 2 in]
            n249 = local read "NM-params"() -> (w575:T2)
            n250 = Index Array(array=w582, index (row) #1=0 ("index (row)"), index (row) #2=1 ("index (row)"), index (row) #3=2 ("index (row)")) -> (element #1=w574:dbl[], element #2=w570:dbl[], element #3=w556:dbl[])  [unwired: 3 in]
            n251 = Unbundle By Name(w575) -> ("sigma"=w571:dbl)
            n252 = Subtract(x=w574, y=w556) -> (x-y=w572:dbl[])
            n253 = Subtract(x=w570, y=w556) -> (x-y=w573:dbl[])
            n254 = Multiply(x=w571, y=w572) -> (x*y=w569:dbl[])
            n255 = Multiply(x=w571, y=w573) -> (x*y=w568:dbl[])
            n256 = Add(x=w569, y=w556) -> (x+y=w567:dbl[])
            n257 = Add(x=w568, y=w556) -> (x+y=w566:dbl[])
            n258 = local read "real-mode"() -> (w558:bool)
            n259 = Build Array(w567, w566) -> (w565:dbl[][])
            n260 = case shown="False" w558 {
              tunnel: w565 -> [w588 w609]
              tunnel: w564 -> [w587 w608]
              tunnel: [w586 w607] -> w561
              tunnel: [w585 w606] -> w560
              frame False {
                n261 = for {
                  shift-right: [w589] -> w586
                  shift-left: w587 -> [w601]
                  tunnel: w588 -> [w594] mode=indexing
                  tunnel: [w593] -> w585 mode=indexing
                  w605 = 1 items=["nearest", "linear", "cubic", "biharmonic spline "] ("method")
                  n262 = Increment(x=w601) -> (x+1=w589:dbl)
                  n263 = Index Array(array=w594, index #1=0 ("index"), index #2=1 ("index")) -> (element #1=w598:dbl, element #2=w596:dbl)
                  n264 = local read "sim-iCorr"() -> (w604:dbl[])
                  n265 = local read "sim-pdx"() -> (w603:dbl[])
                  n266 = local read "sim-pdy"() -> (w602:dbl[])
                  n267 = Build Array(w598) -> (w597:dbl[])
                  n268 = Build Array(w596) -> (w595:dbl[])
                  n269 = call-poly <vilib>:"Interpolate 2D Scattered.vi"("Yi"=w595, "method"=w605, "Xi"=w597, "Y"=w602, "X"=w603, "Z"=w604) -> ("Zi"=w592:dbl[])  [unwired: 4 in, 1 out]
                  n270 = Index Array(array=w592, index=0) -> (element=w591:dbl)
                  n271 = Build Array (concatenate)(w594, w591, w589) -> (w593:dbl[])
                }
              }
              frame True {
                n272 = disable-structure shown="Disabled" {
                  disable-tunnel: w609 -> [w613 _]
                  disable-tunnel: w608 -> [w612 _]
                  disable-tunnel: [w611 _] -> w607
                  disable-tunnel: [w610 _] -> w606
                  frame Disabled {
                    n273 = flat-sequence {
                      tunnel: [w622] -> w610
                      tunnel: [w616] -> w611
                      tunnel: w613 -> [w615]
                      tunnel: w612 -> [w614]
                      frame #0 {
                        n274 = local read "stage-refs"() -> (w618:T1)
                        n275 = local read "stage-error-in"() -> (w619:errorcluster)
                        n276 = local read "meter-error-in"() -> (w617:errorcluster)
                        n277 = Unbundle By Name(w618) -> ("PD X"=w624:refnum<k24>, "PD Y"=w623:refnum<k24>)
                        n278 = for {
                          tunnel: w624 -> [w638]
                          tunnel: w623 -> [w637]
                          tunnel: w615 -> [w634] mode=indexing
                          shift-right: [w632] -> w620
                          shift-left: w619 -> [w636]
                          tunnel: [w635] -> w622 mode=indexing
                          shift-right: [w633] -> w621
                          shift-left: w617 -> [w631]
                          shift-right: [w626] -> w616
                          shift-left: w614 -> [w625]
                          n279 = flat-sequence {
                            tunnel: w638 -> [w649]
                            tunnel: w637 -> [w648]
                            tunnel: w636 -> [w642]
                            tunnel: w634 -> [w640]
                            tunnel: w631 -> [w639]
                            tunnel: [w641] -> w630
                            tunnel: [w640] -> w629
                            tunnel: [w639] -> w628
                            tunnel: [w662] -> w632
                            tunnel: [w658] -> w633
                            tunnel: [w661] -> w635
                            tunnel: w630 -> [w662]
                            tunnel: w629 -> [w660]
                            tunnel: w628 -> [w659]
                            tunnel: w626 -> [w652]
                            frame #0 {
                              w647 = 12000 ("waitTimeout")
                              n280 = Index Array(array=w640, index #1=0 ("index"), index #2=1 ("index")) -> (element #1=w644:dbl, element #2=w643:dbl)
                              n281 = invoke class="IntegratedStepperMotor" method="MoveTo"(reference=w649, "position"=w644, "waitTimeout"=w647) -> (error out=w651:errorcluster)  [unwired: 2 in, 4 out]
                              n282 = invoke class="IntegratedStepperMotor" method="MoveTo"(reference=w648, "position"=w643, "waitTimeout"=w647) -> (error out=w650:errorcluster)  [unwired: 2 in, 4 out]
                              n283 = Merge Errors(w642, w651, w650) -> (w641:errorcluster)
                            }
                            frame #1 {
                              n284 = local read "nSamples"() -> (w657:dbl)
                              n285 = local read "PD Values"() -> (w655:cluster{"PD1":dbl, "PD2":dbl, "PD3":dbl})
                              n286 = local read "meter-visa"() -> (w656:refnum<visa-resource-name>)
                              n287 = call "meter_buffered.vi"("F=cRIO"="F=cRIO 2", "Samples"=w657, "error in"=w659, "PD ranges"=w655, "meter-VISA"=w656) -> ("error out"=w658:errorcluster, "iCorr"=w653:dbl)  [unwired: 2 in, 3 out]
                              n288 = Build Array (concatenate)(w660, w653, w652) -> (w661:dbl[])
                            }
                          }
                          n289 = Increment(x=w625) -> (x+1=w627:dbl)
                          n290 = To Double Precision Float(number=w627) -> (double precision float=w626:dbl)
                        }
                        n291 = local write "stage-error-out"(w620) -> ()
                        n292 = local write "stage-error-out"(w621) -> ()
                      }
                    }
                  }
                  frame Enabled {
                  }
                }
              }
            }
            n293 = Build Array (concatenate)(w560, w556) -> (w557:dbl[][])
            n294 = Build Array (concatenate)(w563, w557) -> (w562:dbl[][])
          }
        }
        n295 = Or(x=w144, y="early-stop") -> (x .or. y?=w145:bool)
        "nPts" <- w151
        "state" <- w154
      }
    }
  }
  "Final Location" <- w7
  "pt-history" <- w6
  "Array" <- w5
